vi "boc_tablo_0_measurment.vi"(8 "error in (no error)":errorcluster, 9 "delay_before_measure":dbl min=0.0, 10 "UI in":T8, 11 "Param_in":T1) -> (0 "error out":errorcluster, 1 "measured_value":dbl[](array[numeric]), 2 "UI out":T8, 3 "Param_out":T1, 4 "DC":dbl[](array[numeric]), 5 "progress":u8(slide) scale=0.0..100.0, 6 "RMS":dbl[](array[numeric]), 7 "plot":waveform(sgl)[](array[waveform]))   [LabVIEW 2017]
uses:
  ui.ctl
  ui_buttons.ctl
  types/boc_type.ctl
  Unicorn Labview Library/Control/unicorn_Param.ctl
  Unicorn Labview Library/Control/unicorn_conn.ctl
  Unicorn Labview Library/Control/unicorn_JSON.ctl
  Unicorn Labview Library/Control/unicorn_ParamInt.ctl
  Unicorn Labview Library/Control/unicorn_Telemetry.ctl
  Unicorn Labview Library/Control/unicorn_Table.ctl
  Unicorn Labview Library/Control/unicorn_ParamFloat.ctl
  Unicorn Labview Library/Unicorn Library.lvlib
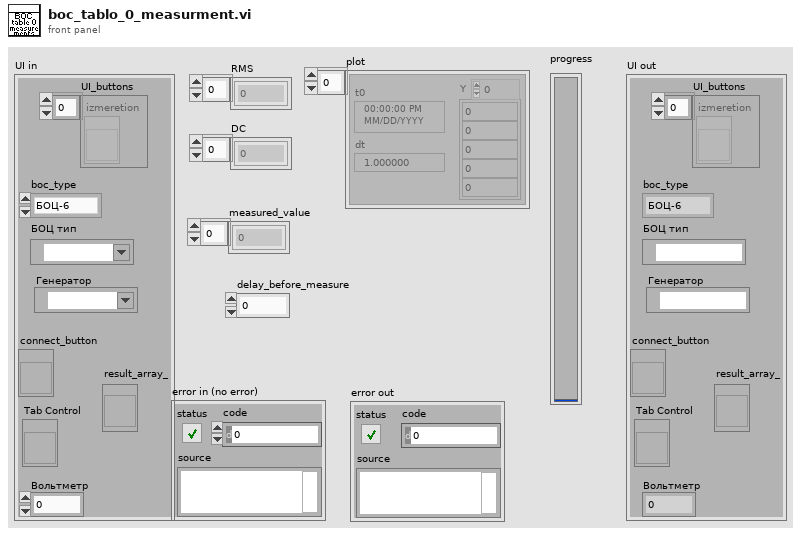
[diagram p1: front panel]
types:
  T1 = typedef "Unicorn Library.lvlib/unicorn_Param.ctl" = cluster{"conParam":T2, "Param":T3}
  T2 = typedef "Unicorn Library.lvlib/unicorn_conn.ctl" = cluster{"ReadIntParam":bool, "ReadDescrParam":bool, "ReadFloatParam":bool, "debug":bool, "ReadJSON":bool, "IP_address":string, "N_attempts":i32, "type_con":enum16{"Serial", "TCP"}, "MB_address":i32, "VISA":refnum<visa-resource-name>, "connection ID":refnum<k5>, "nameDevices":string, "timeout":i32, "port":u16, "type_version":string, "baud_rate":u32, "VersionControl":bool, "TCP_conn":bool, "WindowSize":i32}
  T3 = typedef "Unicorn Library.lvlib/unicorn_JSON.ctl" = cluster{"NumParam":cluster{"NTelem":i32, "NInt":i32, "NFloat":i32, "NTable":i32}, "ParamInt":T4, "Telemetry":T5, "Table":T6, "ParamFloat":T7}
  T4 = typedef "Unicorn Library.lvlib/unicorn_ParamInt.ctl" = cluster{"ID":string, "Num":i32, "Name":string, "Type":string, "Enum":string, "Desc":string, "Unit":string, "Access":string, "FormatStr":string, "Min":i32, "Max":i32}[]
  T5 = typedef "Unicorn Library.lvlib/unicorn_Telemetry.ctl" = cluster{"ID":string, "Num":i32, "Name":string, "Desc":string, "Unit":string, "FormatStr":string, "Min":i32, "Max":i32}[]
  T6 = typedef "Unicorn Library.lvlib/unicorn_Table.ctl" = cluster{"Num":i32, "Access":string, "ColumnCount":i32, "NeedParamPrepare":bool, "Columns":cluster{"Column":i32, "Desc":string, "Name":string}[], "DataType":string, "FormatStr":string, "ID":string, "Name":string, "RowCount":i32, "Rows":cluster{"Desc":string, "ID":string, "Max":i32, "Min":i32, "Name":string, "Row":i32, "Unit":string}[], "Type":string}[]
  T7 = typedef "Unicorn Library.lvlib/unicorn_ParamFloat.ctl" = cluster{"ID":string, "Num":i32, "Name":string, "Type":string, "Enum":string, "Desc":string, "Unit":string, "Access":string, "FormatStr":string, "Min":i32, "Max":i32}[]
  T8 = typedef "ui.ctl" = cluster{"UI_buttons":T9, "Tab Control":refnum<vi>, "connect_button":refnum<vi>, "generator":refnum<visa-resource-name>, "voltmetr":refnum<visa-resource-name>, "channel_timeout_sec":dbl, "boc_type":T10, "result_array_":refnum<vi>}
  T9 = typedef "ui_buttons.ctl" = refnum<vi>[]
  T10 = typedef "boc_type.ctl" = enum16{"БОЦ-6", "БОЦ-12"}
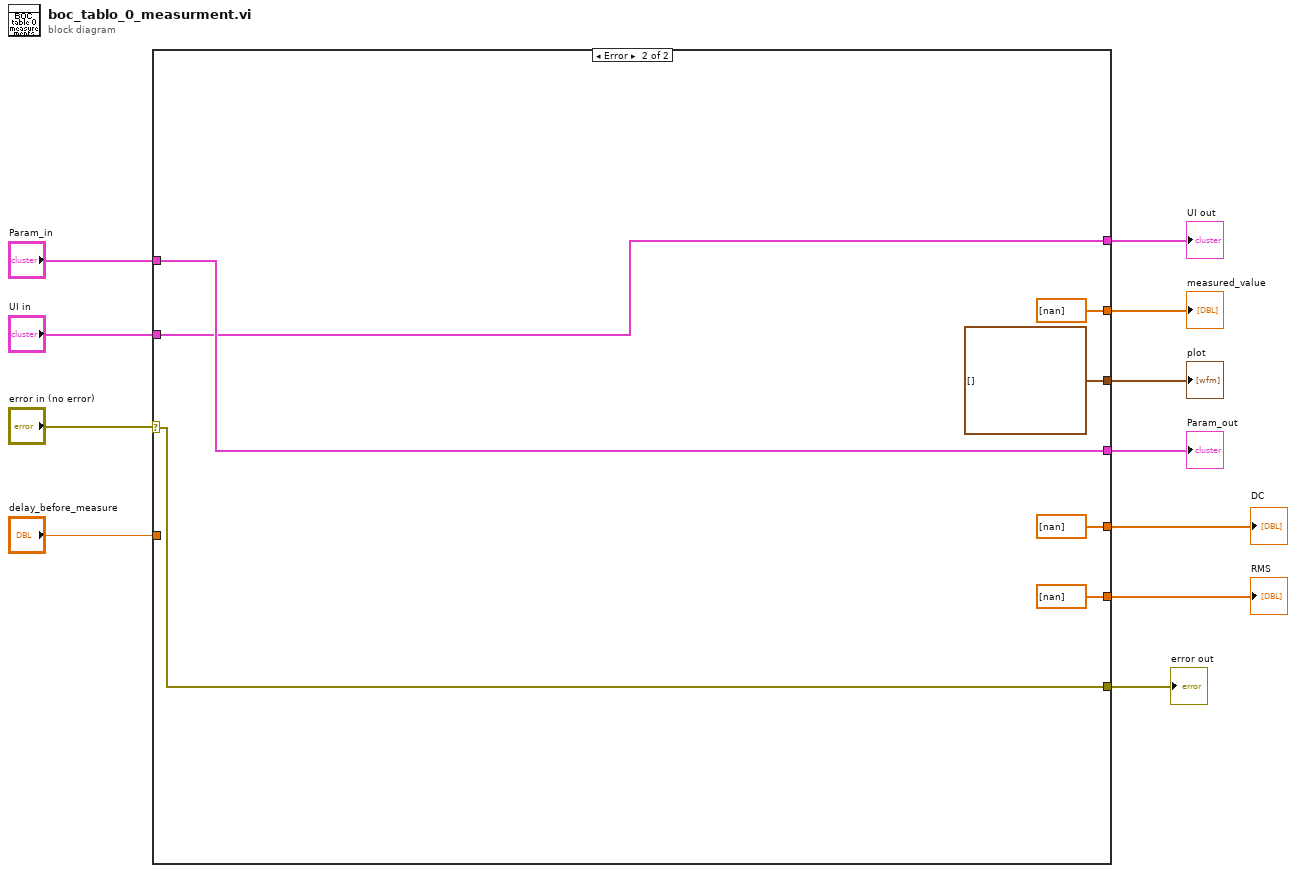
[diagram p0: block diagram]
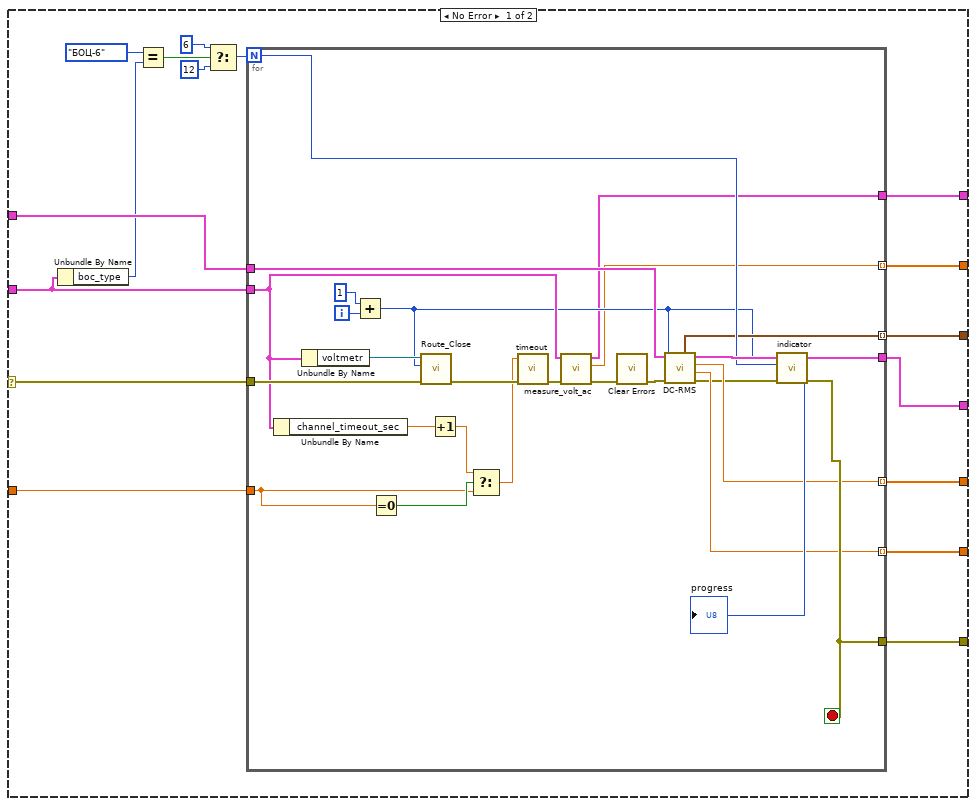
[diagram p2: hidden frame]
diagram:
  n1 = case shown="Error" "error in (no error)" {
    selector: "error in (no error)" -> [w12 w59]
    tunnel: [w28 waveform(sgl)[] []] -> w11
    tunnel: [w27 w59] -> w10
    tunnel: [w26 w61] -> w9
    tunnel: "Param_in" -> [w25 w61]
    tunnel: [w24 dbl[] [nan]] -> w7
    tunnel: "UI in" -> [w18 w60]
    tunnel: [w16 dbl[] [nan]] -> w5
    tunnel: [w15 w60] -> w4
    tunnel: [w14 dbl[] [nan]] -> w3
    tunnel: "delay_before_measure" -> [w13 _]
    frame No Error {
      n2 = Unbundle By Name(w18) -> ("boc_type"=w17:T10)
      n3 = Equal?(x=enum16{"БОЦ-6", "БОЦ-12"}."БОЦ-6", y=w17) -> (x = y?=w20:bool)
      n4 = Select(t=u8 6, s=w20, f=u8 12) -> (s? t:f=w23:u8)
      n5 = for {
        N: w23 -> [w47]
        tunnel: [w38] -> w24 mode=indexing
        tunnel: w12 -> [w52]
        tunnel: w25 -> [w51]
        tunnel: [w50] -> w26
        tunnel: [w48] -> w27
        tunnel: w18 -> [w43]
        tunnel: [w46] -> w28 mode=indexing
        tunnel: [w39] -> w16 mode=indexing
        tunnel: [w37] -> w14 mode=indexing
        tunnel: [w36] -> w15
        tunnel: w13 -> [w32]
        i -> [w41]
        stop <- w48 stop-if-true
        n6 = Unbundle By Name(w43) -> ("channel_timeout_sec"=w45:dbl)
        n7 = Unbundle By Name(w43) -> ("voltmetr"=w49:refnum<visa-resource-name>)
        n8 = Add(x=1, y=w41) -> (x+y=w40:i32)
        n9 = Equal To 0?(x=w32) -> (x = 0?=w35:bool)
        n10 = call <instrlib>:"Route_Close.vi"("error in (no error)"=w52, "channel"=w40, "VISA resource name"=w49) -> ("error out"=w53:errorcluster)  [unwired: 6 in, 2 out]
        n11 = Increment(x=w45) -> (x+1=w34:dbl)
        n12 = Select(t=w34, s=w35, f=w32) -> (s? t:f=w33:dbl)
        n13 = call "timeout.vi"("error in (no error)"=w53, "seconds to wait"=w33) -> ("error IO"=w42:errorcluster)  [unwired: 9 in]
        n14 = call "measure_volt_ac.vi"("error in (no error)"=w42, "UI in in"=w43) -> ("error out"=w29:errorcluster, "Measurement"=w37:dbl, "UI out"=w36:T8)  [unwired: 7 in]
        n15 = call <vilib>:"Clear Errors.vi"("error in (no error)"=w29) -> ("error out"=w30:errorcluster)  [unwired: 5 in, 1 out]
        n16 = call "DC-RMS.vi"("error in (no error)"=w30, "channel"=w40, "ParamIn"=w51) -> ("error out"=w31:errorcluster, "RMS values"=w39:dbl, "DC values"=w38:dbl, "ParamOut"=w50:T1, "Waveform"=w46:waveform(sgl))  [unwired: 4 in]
        n17 = call "indicator.vi"("error_in"=w31, "count"=w47, "current_num"=w40) -> ("error_out"=w48:errorcluster, "Slide"=→"progress":u8)  [unwired: 7 in]
      }
    }
    frame Error {
    }
  }
  "UI out" <- w4
  "plot" <- w11
  "error out" <- w10
  "Param_out" <- w9
  "DC" <- w7
  "RMS" <- w5
  "measured_value" <- w3
